vi "SetPresetSettings.vi"(0 "VISA resource name":refnum<visa-resource-name>, 1 "Voltage":dbl, 2 "Current":dbl, 3 "error in (no error)":errorcluster, 4 "Preset":enum16{"0", "1", "2", "3", ""}(ring)) -> (5 "VISA resource name out":refnum<visa-resource-name>, 6 "error out":errorcluster)   [LabVIEW 2019, in "9103Series.lvlib"]
uses:
  <instrlib>/9103Series/9103Series.lvlib
panel:
  out "ok?":string
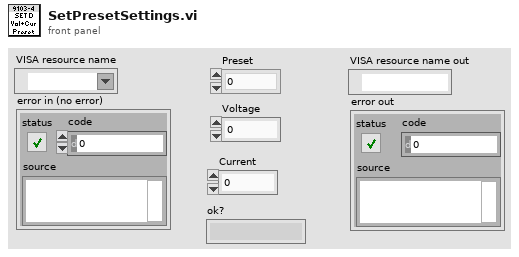
[diagram p1: front panel]
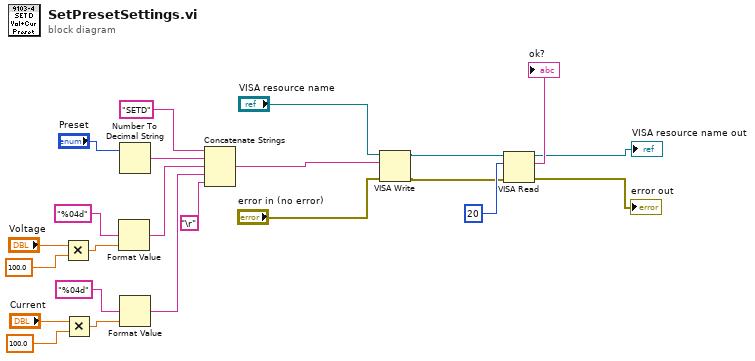
[diagram p0: block diagram]
diagram:
  n1 = Multiply(x="Voltage", y=100.0) -> (x*y=w14:dbl)
  n2 = Multiply(x="Current", y=100.0) -> (x*y=w3:dbl)
  n3 = Format Value(format string="%04d", value (0)=w14) -> (output string=w19:string)  [unwired: 1 in]
  n4 = Number To Decimal String(number="Preset") -> (decimal integer string=w20:string)  [unwired: 1 in]
  n5 = Format Value(format string="%04d", value (0)=w3) -> (output string=w1:string)  [unwired: 1 in]
  n6 = Concatenate Strings("SETD" ("string"), w20, w19, w1, "\r") -> (w17:string)
  n7 = VISA Write(VISA resource name="VISA resource name", write buffer=w17, error in (no error)="error in (no error)") -> (VISA resource name out=w8:refnum<visa-resource-name>, error out=w7:errorcluster)  [unwired: 1 out]
  n8 = VISA Read(VISA resource name=w8, byte count=u32 20, error in (no error)=w7) -> (VISA resource name out=→"VISA resource name out":refnum<visa-resource-name>, read buffer=→"ok?":string, error out=→"error out":errorcluster)  [unwired: 1 out]
